vi "configureCamera.vi"(8 "error in (no error)":errorcluster, 9 "video":bool, 10 "device":string, 11 "AtomChipHWC in":refnum<class "AtomChipHWC.lvclass">) -> (0 "error out":errorcluster, 3 "AtomChipHWC out":refnum<class "AtomChipHWC.lvclass">)   [LabVIEW 2011, in "Hardware.lvlib" / "HWControllers.lvlib" / "AtomChipHWC.lvclass"]
uses:
  AtomChipHWC.lvclass
  AtomChipHWC.lvclass/AtomChipHWC.ctl
  Tools/Filing/FileSystem/FileSystem.lvclass
  Network Controllers/NetworkCamera/NetworkCamera.lvclass
  Tools/CameraSettings/CamaraSettings.lvclass
  HWController.lvclass
  Network Controllers/CameraNetworkController/CameraNetworkController.lvclass
  Tools/Filing/FileNeologist/FileNeologist.lvclass
  Tools/Filing.lvlib
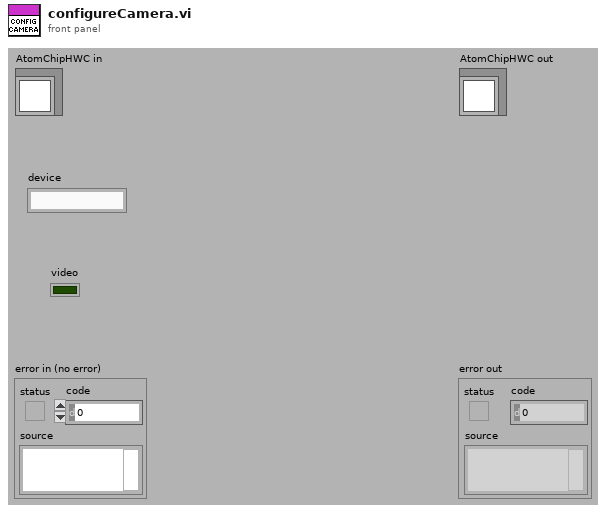
[diagram p1: front panel]
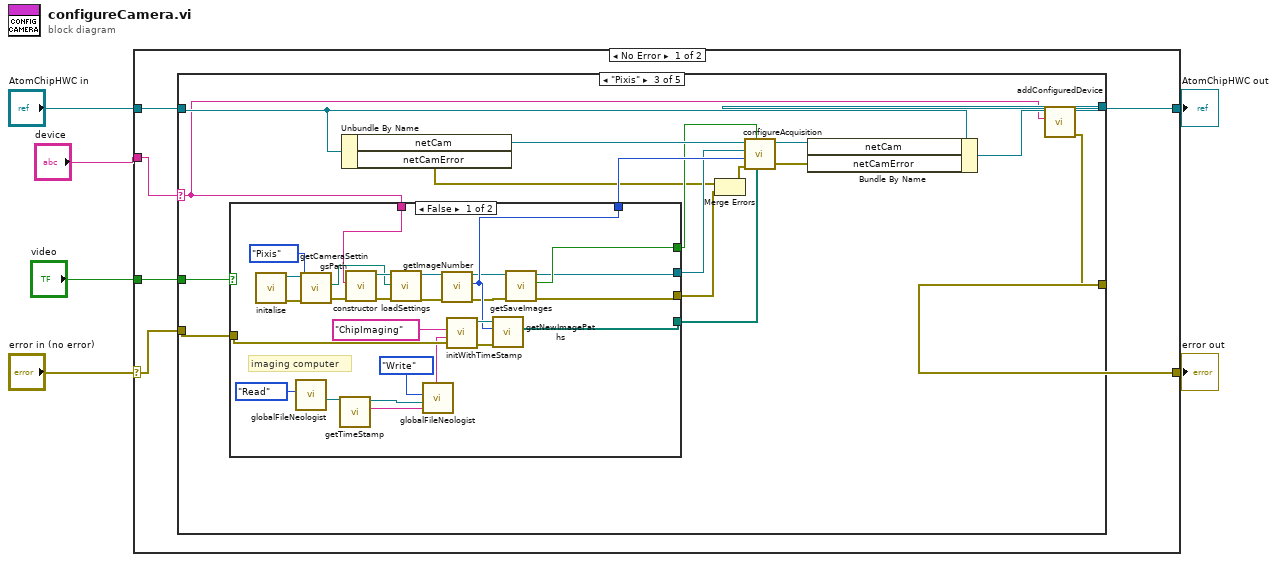
[diagram p0: block diagram]
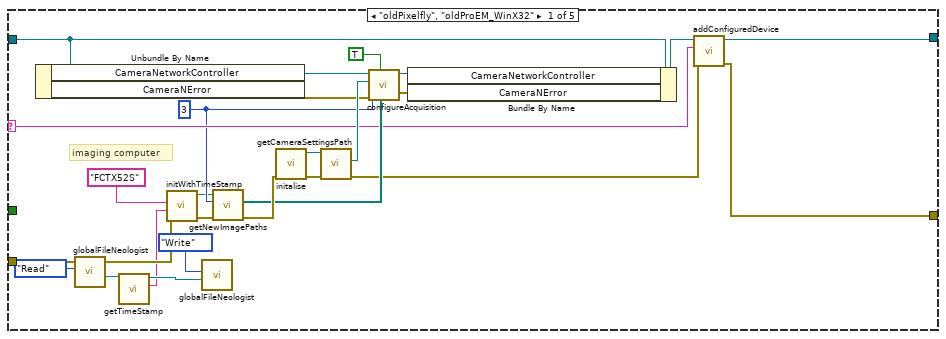
[diagram p2: hidden frame]
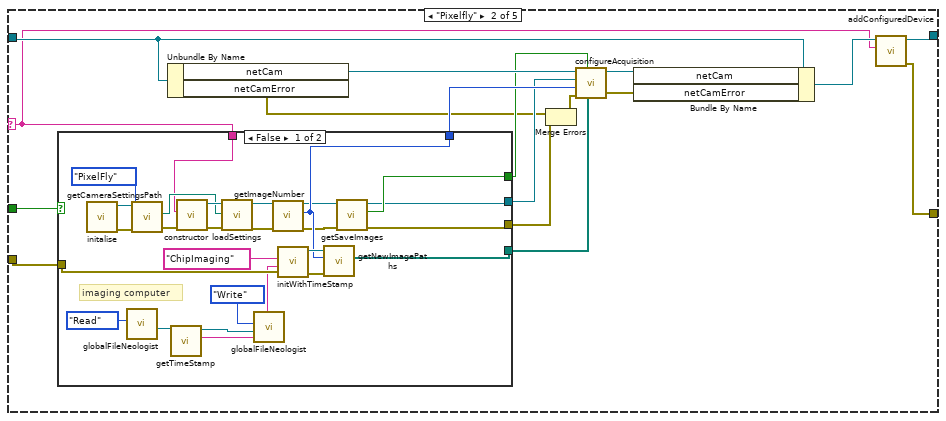
[diagram p3: hidden frame]
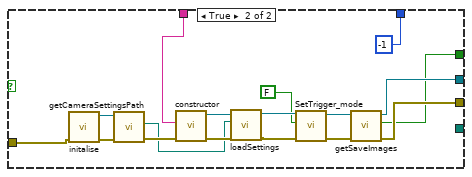
[diagram p4: hidden frame]
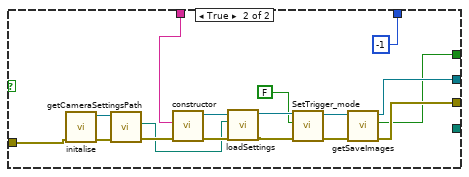
[diagram p5: hidden frame]
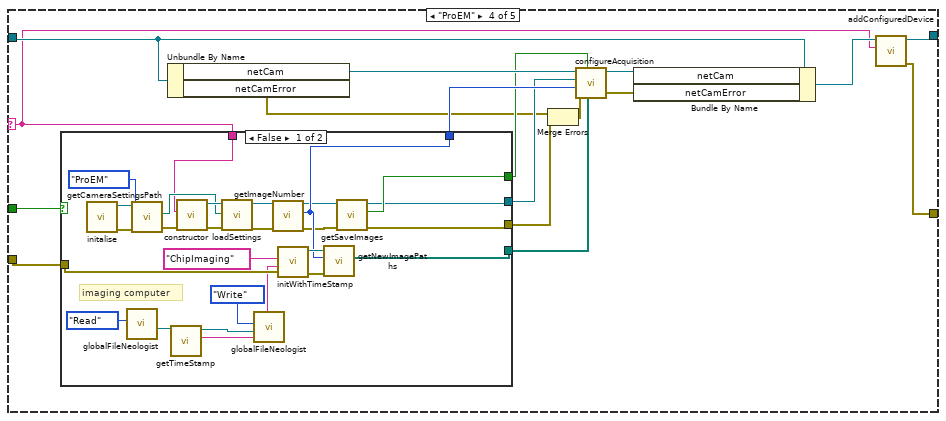
[diagram p6: hidden frame]
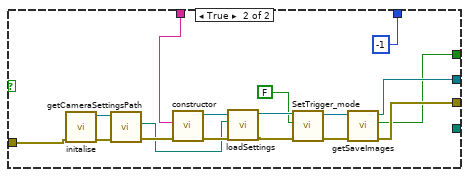
[diagram p7: hidden frame]
diagram:
  n1 = case shown="No Error" "error in (no error)" {
    selector: "error in (no error)" -> [w11 w222]
    tunnel: [w10 w222] -> w5
    tunnel: [w12 w221] -> w3
    tunnel: "AtomChipHWC in" -> [w9 w221]
    tunnel: "device" -> [w8 _]
    tunnel: "video" -> [w7 _]
    frame No Error {
      n2 = case shown="\"Pixis\"" w8 {
        selector: w8 -> [w27 w45 w105 w165 _]
        tunnel: [w28 w53 w113 w173 w220] -> w12
        tunnel: w11 -> [w22 w51 w111 w171 w219]
        tunnel: [w26 w52 w112 w172 w219] -> w10
        tunnel: w9 -> [w37 w55 w115 w175 w220]
        tunnel: w7 -> [_ w42 w102 w162 _]
        frame "oldPixelfly", "oldProEM_WinX32" {
          w25 = 3
          # "imaging computer"
          n3 = Unbundle By Name(w37) -> ("CameraNetworkController"=w38:refnum<class "CameraNetworkController.lvclass">, "CameraNError"=w15:errorcluster)
          n4 = call "globalFileNeologist.vi"("Action"=enum16{"Write", "Read"}."Read") -> ("FileNeologist out"=w18:refnum<class "FileNeologist.lvclass">)  [unwired: 10 in]
          n5 = call "getTimeStamp.vi"("FileNeologist in"=w18) -> ("TimeStamp"=w16:string, "FileNeologist out"=w17:refnum<class "FileNeologist.lvclass">)  [unwired: 8 in, 1 out]
          n6 = call "initWithTimeStamp.vi"("error in (no error)"=w22, "timeStamp"=w16, "computer name"="FCTX52S") -> ("error out"=w24:errorcluster, "FileNeologist out"=w23:refnum<class "FileNeologist.lvclass">)  [unwired: 7 in]
          n7 = call "globalFileNeologist.vi"("FileNeologist in"=w17, "Action"=enum16{"Write", "Read"}."Write") -> ()  [unwired: 9 in, 1 out]
          n8 = call "getNewImagePaths.vi"("error in (no error)"=w24, "numberOfImages"=w25, "FileNeologist in"=w23) -> ("error out"=w31:errorcluster, "Paths"=w30:path[])  [unwired: 6 in, 1 out]
          n9 = call "initalise.vi"("error in (no error)"=w31) -> ("error out"=w33:errorcluster, "FileSystem out"=w34:refnum<class "FileSystem.lvclass">)  [unwired: 9 in]
          n10 = call-dynamic "getCameraSettingsPath.vi"("error in (no error)"=w33, "FileSystem.lvclass in"=w34) -> ("error out"=w13:errorcluster, "CameraSettingsPath"=w32:path)  [unwired: 7 in, 1 out]
          n11 = call "configureAcquisition.vi"("imagePaths"=w30, "save?"=TRUE, "error in (no error)"=w15, "numberImages"=w25, "settingsPath"=w32, "CameraNetworkController in"=w38) -> ("error out"=w14:errorcluster, "CameraNetworkController out"=w36:refnum<class "CameraNetworkController.lvclass">)  [unwired: 4 in]
          n12 = Bundle By Name(cluster=w37, "CameraNetworkController"=w36, "CameraNError"=w14) -> (w29:refnum<class "AtomChipHWC.lvclass">)
          n13 = call "addConfiguredDevice.vi"("error in (no error)"=w13, "deviceName"=w27, "HWController in"=w29) -> ("error out"=w26:errorcluster, "HWController out"=w28:refnum<class "AtomChipHWC.lvclass">)  [unwired: 7 in]
        }
        frame "Pixelfly" {
          n14 = case shown="False" w42 {
            tunnel: w51 -> [w77 w90]
            tunnel: [w62 -1] -> w48
            tunnel: [w70 _] -> w46
            tunnel: w45 -> [w65 w92]
            tunnel: [w57 w84] -> w44
            tunnel: [w59 w83] -> w39
            tunnel: [w58 w82] -> w43
            frame False {
              # "imaging computer"
              n15 = call "initalise.vi"() -> ("error out"=w80:errorcluster, "FileSystem out"=w81:refnum<class "FileSystem.lvclass">)  [unwired: 10 in]
              n16 = call "globalFileNeologist.vi"("Action"=enum16{"Write", "Read"}."Read") -> ("FileNeologist out"=w73:refnum<class "FileNeologist.lvclass">)  [unwired: 10 in]
              n17 = call-dynamic "getCameraSettingsPath.vi"("error in (no error)"=w80, "Camera"=enum16{"Pixis", "ProEM", "PixelFly"}."PixelFly", "FileSystem.lvclass in"=w81) -> ("error out"=w68:errorcluster, "CameraSettingsPath"=w67:path)  [unwired: 6 in, 1 out]
              n18 = call "getTimeStamp.vi"("FileNeologist in"=w73) -> ("TimeStamp"=w71:string, "FileNeologist out"=w72:refnum<class "FileNeologist.lvclass">)  [unwired: 8 in, 1 out]
              n19 = call "constructor.vi"("error in (no error)"=w68, "camera settings"=w65) -> ("error out"=w66:errorcluster, "CamaraSettings out"=w69:refnum<class "CamaraSettings.lvclass">)  [unwired: 8 in]
              n20 = call-dynamic "loadSettings.vi"("error in (no error)"=w66, "Path"=w67, "CamaraSettings in"=w69) -> ("error out"=w63:errorcluster, "CamaraSettings out"=w64:refnum<class "CamaraSettings.lvclass">)  [unwired: 7 in]
              n21 = call "globalFileNeologist.vi"("FileNeologist in"=w72, "Action"=enum16{"Write", "Read"}."Write") -> ()  [unwired: 9 in, 1 out]
              n22 = call-dynamic "getImageNumber.vi"("error in (no error)"=w63, "CamaraSettings in"=w64) -> ("error out"=w60:errorcluster, "image number"=w62:i32, "CamaraSettings out"=w61:refnum<class "CamaraSettings.lvclass">)  [unwired: 7 in]
              n23 = call "initWithTimeStamp.vi"("error in (no error)"=w77, "timeStamp"=w71, "computer name"="ChipImaging") -> ("error out"=w79:errorcluster, "FileNeologist out"=w78:refnum<class "FileNeologist.lvclass">)  [unwired: 7 in]
              n24 = call "getNewImagePaths.vi"("error in (no error)"=w79, "numberOfImages"=w62, "FileNeologist in"=w78) -> ("Paths"=w70:path[])  [unwired: 6 in, 2 out]
              n25 = call "getSaveImages.vi"("error in (no error)"=w60, "CamaraSettings in"=w61) -> ("error out"=w59:errorcluster, "saveImages"=w58:bool, "CamaraSettings out"=w57:refnum<class "CamaraSettings.lvclass">)  [unwired: 7 in]
            }
            frame True {
              n26 = call "initalise.vi"("error in (no error)"=w90) -> ("error out"=w96:errorcluster, "FileSystem out"=w97:refnum<class "FileSystem.lvclass">)  [unwired: 9 in]
              n27 = call-dynamic "getCameraSettingsPath.vi"("error in (no error)"=w96, "FileSystem.lvclass in"=w97) -> ("error out"=w94:errorcluster, "CameraSettingsPath"=w91:path)  [unwired: 7 in, 1 out]
              n28 = call "constructor.vi"("error in (no error)"=w94, "camera settings"=w92) -> ("error out"=w93:errorcluster, "CamaraSettings out"=w95:refnum<class "CamaraSettings.lvclass">)  [unwired: 8 in]
              n29 = call-dynamic "loadSettings.vi"("error in (no error)"=w93, "Path"=w91, "CamaraSettings in"=w95) -> ("error out"=w88:errorcluster, "CamaraSettings out"=w89:refnum<class "CamaraSettings.lvclass">)  [unwired: 7 in]
              n30 = call-dynamic "SetTrigger_mode.vi"("error in (no error)"=w88, "trigger_mode"=FALSE, "CamaraSettings in"=w89) -> ("error out"=w85:errorcluster, "CamaraSettings out"=w86:refnum<class "CamaraSettings.lvclass">)  [unwired: 7 in]
              n31 = call "getSaveImages.vi"("error in (no error)"=w85, "CamaraSettings in"=w86) -> ("error out"=w83:errorcluster, "saveImages"=w82:bool, "CamaraSettings out"=w84:refnum<class "CamaraSettings.lvclass">)  [unwired: 7 in]
            }
          }
          n32 = Unbundle By Name(w55) -> ("netCam"=w50:refnum<class "NetworkCamera.lvclass">, "netCamError"=w40:errorcluster)
          n33 = Merge Errors(w40, w39) -> (w41:errorcluster)
          n34 = call-dynamic "configureAcquisition.vi"("imagePaths"=w46, "saveImages?"=w43, "error in (no error)"=w41, "number of Images"=w48, "CamaraSettings"=w44, "NetworkCamera in"=w50) -> ("error out"=w47:errorcluster, "NetworkCamera out"=w49:refnum<class "NetworkCamera.lvclass">)  [unwired: 4 in]
          n35 = Bundle By Name(cluster=w55, "netCam"=w49, "netCamError"=w47) -> (w54:refnum<class "AtomChipHWC.lvclass">)
          n36 = call "addConfiguredDevice.vi"("deviceName"=w45, "HWController in"=w54) -> ("error out"=w52:errorcluster, "HWController out"=w53:refnum<class "AtomChipHWC.lvclass">)  [unwired: 8 in]
        }
        frame "Pixis" {
          n37 = case shown="False" w102 {
            tunnel: w111 -> [w137 w150]
            tunnel: [w122 -1] -> w108
            tunnel: [w130 _] -> w106
            tunnel: w105 -> [w125 w152]
            tunnel: [w117 w144] -> w104
            tunnel: [w119 w143] -> w99
            tunnel: [w118 w142] -> w103
            frame False {
              # "imaging computer"
              n38 = call "initalise.vi"() -> ("error out"=w140:errorcluster, "FileSystem out"=w141:refnum<class "FileSystem.lvclass">)  [unwired: 10 in]
              n39 = call "globalFileNeologist.vi"("Action"=enum16{"Write", "Read"}."Read") -> ("FileNeologist out"=w133:refnum<class "FileNeologist.lvclass">)  [unwired: 10 in]
              n40 = call-dynamic "getCameraSettingsPath.vi"("error in (no error)"=w140, "Camera"=enum16{"Pixis", "ProEM", "PixelFly"}."Pixis", "FileSystem.lvclass in"=w141) -> ("error out"=w128:errorcluster, "CameraSettingsPath"=w127:path)  [unwired: 6 in, 1 out]
              n41 = call "getTimeStamp.vi"("FileNeologist in"=w133) -> ("TimeStamp"=w131:string, "FileNeologist out"=w132:refnum<class "FileNeologist.lvclass">)  [unwired: 8 in, 1 out]
              n42 = call "constructor.vi"("error in (no error)"=w128, "camera settings"=w125) -> ("error out"=w126:errorcluster, "CamaraSettings out"=w129:refnum<class "CamaraSettings.lvclass">)  [unwired: 8 in]
              n43 = call-dynamic "loadSettings.vi"("error in (no error)"=w126, "Path"=w127, "CamaraSettings in"=w129) -> ("error out"=w123:errorcluster, "CamaraSettings out"=w124:refnum<class "CamaraSettings.lvclass">)  [unwired: 7 in]
              n44 = call "globalFileNeologist.vi"("FileNeologist in"=w132, "Action"=enum16{"Write", "Read"}."Write") -> ()  [unwired: 9 in, 1 out]
              n45 = call-dynamic "getImageNumber.vi"("error in (no error)"=w123, "CamaraSettings in"=w124) -> ("error out"=w120:errorcluster, "image number"=w122:i32, "CamaraSettings out"=w121:refnum<class "CamaraSettings.lvclass">)  [unwired: 7 in]
              n46 = call "initWithTimeStamp.vi"("error in (no error)"=w137, "timeStamp"=w131, "computer name"="ChipImaging") -> ("error out"=w139:errorcluster, "FileNeologist out"=w138:refnum<class "FileNeologist.lvclass">)  [unwired: 7 in]
              n47 = call "getNewImagePaths.vi"("error in (no error)"=w139, "numberOfImages"=w122, "FileNeologist in"=w138) -> ("Paths"=w130:path[])  [unwired: 6 in, 2 out]
              n48 = call "getSaveImages.vi"("error in (no error)"=w120, "CamaraSettings in"=w121) -> ("error out"=w119:errorcluster, "saveImages"=w118:bool, "CamaraSettings out"=w117:refnum<class "CamaraSettings.lvclass">)  [unwired: 7 in]
            }
            frame True {
              n49 = call "initalise.vi"("error in (no error)"=w150) -> ("error out"=w156:errorcluster, "FileSystem out"=w157:refnum<class "FileSystem.lvclass">)  [unwired: 9 in]
              n50 = call-dynamic "getCameraSettingsPath.vi"("error in (no error)"=w156, "FileSystem.lvclass in"=w157) -> ("error out"=w154:errorcluster, "CameraSettingsPath"=w151:path)  [unwired: 7 in, 1 out]
              n51 = call "constructor.vi"("error in (no error)"=w154, "camera settings"=w152) -> ("error out"=w153:errorcluster, "CamaraSettings out"=w155:refnum<class "CamaraSettings.lvclass">)  [unwired: 8 in]
              n52 = call-dynamic "loadSettings.vi"("error in (no error)"=w153, "Path"=w151, "CamaraSettings in"=w155) -> ("error out"=w148:errorcluster, "CamaraSettings out"=w149:refnum<class "CamaraSettings.lvclass">)  [unwired: 7 in]
              n53 = call-dynamic "SetTrigger_mode.vi"("error in (no error)"=w148, "trigger_mode"=FALSE, "CamaraSettings in"=w149) -> ("error out"=w145:errorcluster, "CamaraSettings out"=w146:refnum<class "CamaraSettings.lvclass">)  [unwired: 7 in]
              n54 = call "getSaveImages.vi"("error in (no error)"=w145, "CamaraSettings in"=w146) -> ("error out"=w143:errorcluster, "saveImages"=w142:bool, "CamaraSettings out"=w144:refnum<class "CamaraSettings.lvclass">)  [unwired: 7 in]
            }
          }
          n55 = Unbundle By Name(w115) -> ("netCam"=w110:refnum<class "NetworkCamera.lvclass">, "netCamError"=w100:errorcluster)
          n56 = Merge Errors(w100, w99) -> (w101:errorcluster)
          n57 = call-dynamic "configureAcquisition.vi"("imagePaths"=w106, "saveImages?"=w103, "error in (no error)"=w101, "number of Images"=w108, "CamaraSettings"=w104, "NetworkCamera in"=w110) -> ("error out"=w107:errorcluster, "NetworkCamera out"=w109:refnum<class "NetworkCamera.lvclass">)  [unwired: 4 in]
          n58 = Bundle By Name(cluster=w115, "netCam"=w109, "netCamError"=w107) -> (w114:refnum<class "AtomChipHWC.lvclass">)
          n59 = call "addConfiguredDevice.vi"("deviceName"=w105, "HWController in"=w114) -> ("error out"=w112:errorcluster, "HWController out"=w113:refnum<class "AtomChipHWC.lvclass">)  [unwired: 8 in]
        }
        frame "ProEM" {
          n60 = case shown="False" w162 {
            tunnel: w171 -> [w197 w210]
            tunnel: [w182 -1] -> w168
            tunnel: [w190 _] -> w166
            tunnel: w165 -> [w185 w212]
            tunnel: [w177 w204] -> w164
            tunnel: [w179 w203] -> w159
            tunnel: [w178 w202] -> w163
            frame False {
              # "imaging computer"
              n61 = call "initalise.vi"() -> ("error out"=w200:errorcluster, "FileSystem out"=w201:refnum<class "FileSystem.lvclass">)  [unwired: 10 in]
              n62 = call "globalFileNeologist.vi"("Action"=enum16{"Write", "Read"}."Read") -> ("FileNeologist out"=w193:refnum<class "FileNeologist.lvclass">)  [unwired: 10 in]
              n63 = call-dynamic "getCameraSettingsPath.vi"("error in (no error)"=w200, "Camera"=enum16{"Pixis", "ProEM", "PixelFly"}."ProEM", "FileSystem.lvclass in"=w201) -> ("error out"=w188:errorcluster, "CameraSettingsPath"=w187:path)  [unwired: 6 in, 1 out]
              n64 = call "getTimeStamp.vi"("FileNeologist in"=w193) -> ("TimeStamp"=w191:string, "FileNeologist out"=w192:refnum<class "FileNeologist.lvclass">)  [unwired: 8 in, 1 out]
              n65 = call "constructor.vi"("error in (no error)"=w188, "camera settings"=w185) -> ("error out"=w186:errorcluster, "CamaraSettings out"=w189:refnum<class "CamaraSettings.lvclass">)  [unwired: 8 in]
              n66 = call-dynamic "loadSettings.vi"("error in (no error)"=w186, "Path"=w187, "CamaraSettings in"=w189) -> ("error out"=w183:errorcluster, "CamaraSettings out"=w184:refnum<class "CamaraSettings.lvclass">)  [unwired: 7 in]
              n67 = call "globalFileNeologist.vi"("FileNeologist in"=w192, "Action"=enum16{"Write", "Read"}."Write") -> ()  [unwired: 9 in, 1 out]
              n68 = call-dynamic "getImageNumber.vi"("error in (no error)"=w183, "CamaraSettings in"=w184) -> ("error out"=w180:errorcluster, "image number"=w182:i32, "CamaraSettings out"=w181:refnum<class "CamaraSettings.lvclass">)  [unwired: 7 in]
              n69 = call "initWithTimeStamp.vi"("error in (no error)"=w197, "timeStamp"=w191, "computer name"="ChipImaging") -> ("error out"=w199:errorcluster, "FileNeologist out"=w198:refnum<class "FileNeologist.lvclass">)  [unwired: 7 in]
              n70 = call "getNewImagePaths.vi"("error in (no error)"=w199, "numberOfImages"=w182, "FileNeologist in"=w198) -> ("Paths"=w190:path[])  [unwired: 6 in, 2 out]
              n71 = call "getSaveImages.vi"("error in (no error)"=w180, "CamaraSettings in"=w181) -> ("error out"=w179:errorcluster, "saveImages"=w178:bool, "CamaraSettings out"=w177:refnum<class "CamaraSettings.lvclass">)  [unwired: 7 in]
            }
            frame True {
              n72 = call "initalise.vi"("error in (no error)"=w210) -> ("error out"=w216:errorcluster, "FileSystem out"=w217:refnum<class "FileSystem.lvclass">)  [unwired: 9 in]
              n73 = call-dynamic "getCameraSettingsPath.vi"("error in (no error)"=w216, "FileSystem.lvclass in"=w217) -> ("error out"=w214:errorcluster, "CameraSettingsPath"=w211:path)  [unwired: 7 in, 1 out]
              n74 = call "constructor.vi"("error in (no error)"=w214, "camera settings"=w212) -> ("error out"=w213:errorcluster, "CamaraSettings out"=w215:refnum<class "CamaraSettings.lvclass">)  [unwired: 8 in]
              n75 = call-dynamic "loadSettings.vi"("error in (no error)"=w213, "Path"=w211, "CamaraSettings in"=w215) -> ("error out"=w208:errorcluster, "CamaraSettings out"=w209:refnum<class "CamaraSettings.lvclass">)  [unwired: 7 in]
              n76 = call-dynamic "SetTrigger_mode.vi"("error in (no error)"=w208, "trigger_mode"=FALSE, "CamaraSettings in"=w209) -> ("error out"=w205:errorcluster, "CamaraSettings out"=w206:refnum<class "CamaraSettings.lvclass">)  [unwired: 7 in]
              n77 = call "getSaveImages.vi"("error in (no error)"=w205, "CamaraSettings in"=w206) -> ("error out"=w203:errorcluster, "saveImages"=w202:bool, "CamaraSettings out"=w204:refnum<class "CamaraSettings.lvclass">)  [unwired: 7 in]
            }
          }
          n78 = Unbundle By Name(w175) -> ("netCam"=w170:refnum<class "NetworkCamera.lvclass">, "netCamError"=w160:errorcluster)
          n79 = Merge Errors(w160, w159) -> (w161:errorcluster)
          n80 = call-dynamic "configureAcquisition.vi"("imagePaths"=w166, "saveImages?"=w163, "error in (no error)"=w161, "number of Images"=w168, "CamaraSettings"=w164, "NetworkCamera in"=w170) -> ("error out"=w167:errorcluster, "NetworkCamera out"=w169:refnum<class "NetworkCamera.lvclass">)  [unwired: 4 in]
          n81 = Bundle By Name(cluster=w175, "netCam"=w169, "netCamError"=w167) -> (w174:refnum<class "AtomChipHWC.lvclass">)
          n82 = call "addConfiguredDevice.vi"("deviceName"=w165, "HWController in"=w174) -> ("error out"=w172:errorcluster, "HWController out"=w173:refnum<class "AtomChipHWC.lvclass">)  [unwired: 8 in]
        }
        frame Default {
        }
      }
    }
    frame Error {
    }
  }
  "error out" <- w5
  "AtomChipHWC out" <- w3
